vi "Read Transconductance (Voltage).vi"(0 "VISA resource name":refnum<visa-resource-name>, 1 "Pulse Stop Level (0.1 V)":dbl=0.1, 2 "Pulse Start Level (0 V)":dbl, 5 "Source Measure Unit Channel (0: Channel A)":i32(ring) items=["Channel A", "Channel B"], 7 "Current Buffer (ibuffer)":string="ibuffer", 9 "Voltage Buffer (vbuffer)":string="vbuffer", 11 "error in (no error)":errorcluster, 12 "Pulse Measure Cycles (10)":i32=10) -> (4 "VISA resource name out":refnum<visa-resource-name>, 6 "Transconductance":dbl[](array[numeric]), 8 "Current (A)":dbl[](array[numeric]), 10 "Voltage (V)":dbl[](array[numeric]), 15 "error out":errorcluster)   [LabVIEW 2015, in "Keithley 2600 Series.lvlib"]
doc: "Performs a linear voltage sweep and calculates the transconductance.\n\n<b>Note:</b>\nThere are three options for the measurements during the voltage sweep: transconductance measurement; transconductance and current measurement; transconductance, voltage and current measurement."
uses:
  Keithley 2600 Series.lvlib
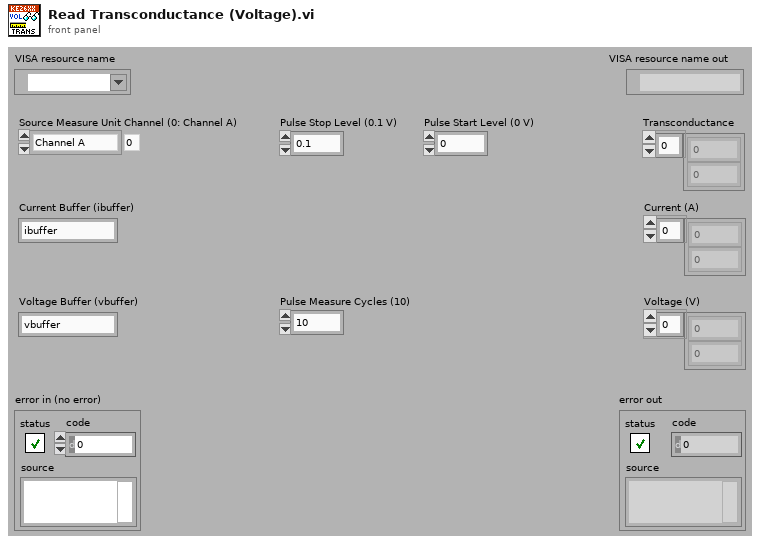
[diagram p1: front panel]
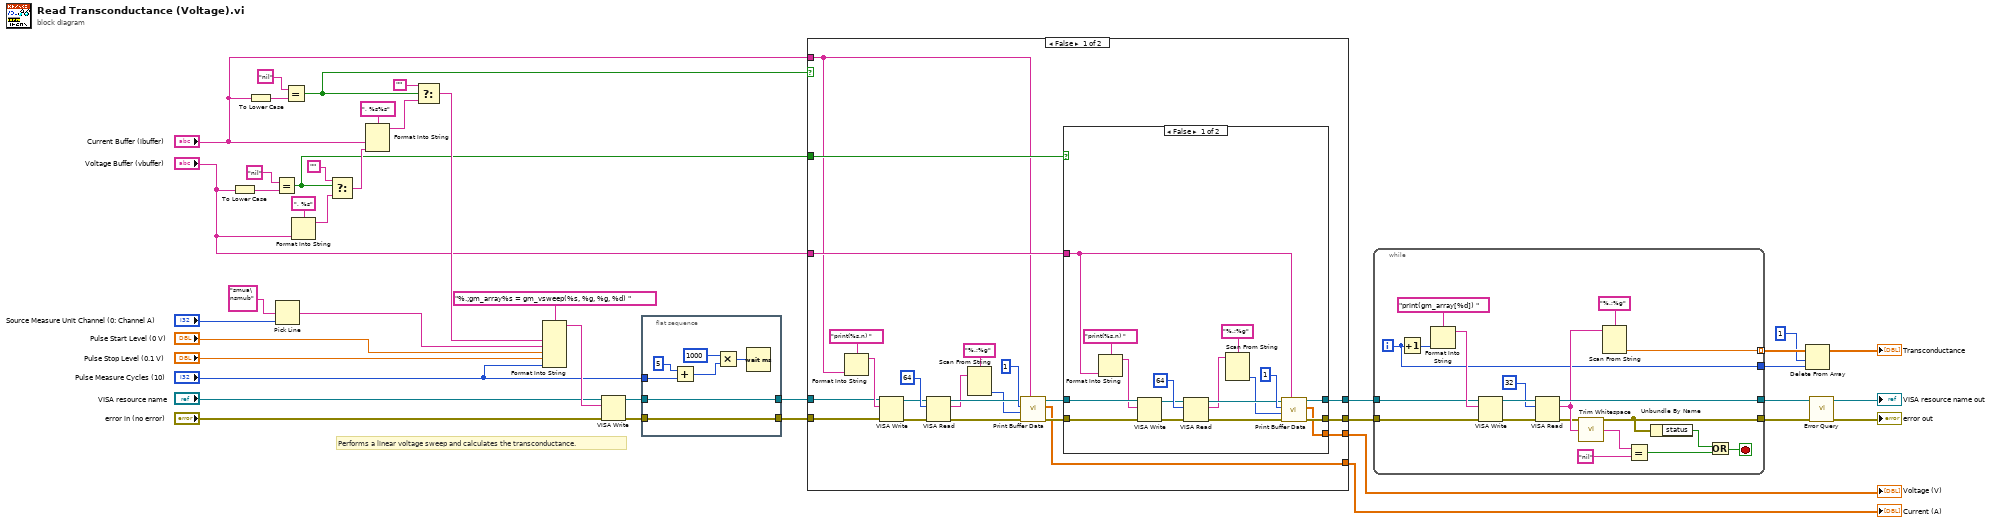
[diagram p0: block diagram]
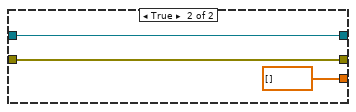
[diagram p2: hidden frame]
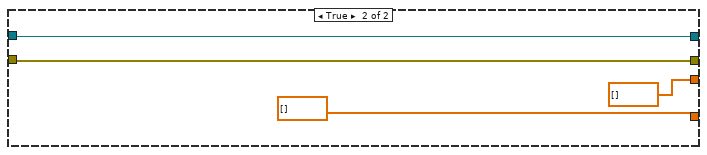
[diagram p3: hidden frame]
diagram:
  # "Performs a linear voltage sweep and calculates the transconductance."
  n1 = To Lower Case(string="Voltage Buffer (vbuffer)") -> (all lower case string=w7:string)
  n2 = To Lower Case(string="Current Buffer (ibuffer)") -> (all lower case string=w9:string)
  n3 = Equal?(x="nil", y=w7) -> (x = y?=w27:bool)
  n4 = Pick Line(multi-line string="smua\nsmub", line index="Source Measure Unit Channel (0: Channel A)") -> (output string=w29:string)  [unwired: 1 in]
  n5 = Equal?(x="nil", y=w9) -> (x = y?=w28:bool)
  n6 = Format Into String(format string=", %s", "Voltage Buffer (vbuffer)") -> (resulting string=w33:string)  [unwired: 2 in, 1 out]
  n7 = Select(t="", s=w27, f=w33) -> (s? t:f=w32:string)
  n8 = Format Into String(format string=", %s%s", "Current Buffer (ibuffer)", w32) -> (resulting string=w31:string)  [unwired: 2 in, 1 out]
  n9 = Select(t="", s=w28, f=w31) -> (s? t:f=w30:string)
  n10 = Format Into String(format string="%.;gm_array%s = gm_vsweep(%s, %g, %g, %d) ", w30, w29, "Pulse Start Level (0 V)", "Pulse Stop Level (0.1 V)", "Pulse Measure Cycles (10)") -> (resulting string=w41:string)  [unwired: 2 in, 1 out]
  n11 = VISA Write(VISA resource name="VISA resource name", write buffer=w41, error in (no error)="error in (no error)") -> (VISA resource name out=w13:refnum<visa-resource-name>, error out=w12:errorcluster)  [unwired: 1 out]
  n12 = flat-sequence {
    tunnel: w13 -> [w49]
    tunnel: w12 -> [w48]
    tunnel: [w49] -> w11
    tunnel: [w48] -> w10
    tunnel: "Pulse Measure Cycles (10)" -> [w46]
    frame #0 {
      n13 = Add(x=5, y=w46) -> (x+y=w44:i32)
      n14 = Multiply(x=1000 ("y"), y=w44) -> (x*y=w43:i32)
      n15 = Wait (ms)(milliseconds to wait=w43) -> ()  [unwired: 1 out]
    }
  }
  n16 = case shown="False" w28 {
    tunnel: [w56 w95] -> w26
    tunnel: w11 -> [w60 w95]
    tunnel: w10 -> [w59 w94]
    tunnel: [w55 w94] -> w25
    tunnel: w27 -> [w54 _]
    tunnel: "Voltage Buffer (vbuffer)" -> [w53 _]
    tunnel: [w52 dbl[] [] ("Buffer Data")] -> w15
    tunnel: [w51 dbl[] [] ("Buffer Data")] -> w14
    tunnel: "Current Buffer (ibuffer)" -> [w50 _]
    frame False {
      n17 = Format Into String(format string="print(%s.n) ", w50) -> (resulting string=w61:string)  [unwired: 2 in, 1 out]
      n18 = VISA Write(VISA resource name=w60, write buffer=w61, error in (no error)=w59) -> (VISA resource name out=w64:refnum<visa-resource-name>, error out=w63:errorcluster)  [unwired: 1 out]
      n19 = VISA Read(VISA resource name=w64, byte count=u32 64, error in (no error)=w63) -> (VISA resource name out=w69:refnum<visa-resource-name>, read buffer=w67:string, error out=w68:errorcluster)  [unwired: 1 out]
      n20 = Scan From String(format string="%.;%g", input string=w67) -> (output 1=w66:i32)  [unwired: 3 in, 3 out]
      n21 = call "Print Buffer Data.vi"("Reading Buffer (smua.nvbuffer1)"=w50, "error in (no error)"=w68, "End Index (1)"=w66, "Start Index (1)"=1 ("Start Index (0)"), "VISA resource name"=w69) -> ("error out"=w57:errorcluster, "Buffer Data"=w52:dbl[], "VISA resource name out"=w58:refnum<visa-resource-name>)  [unwired: 4 in]
      n22 = case shown="False" w54 {
        tunnel: w58 -> [w80 w91]
        tunnel: w57 -> [w79 w90]
        tunnel: [w78 w91] -> w56
        tunnel: [w77 w90] -> w55
        tunnel: w53 -> [w74 _]
        tunnel: [w73 dbl[] [] ("Buffer Data")] -> w51
        frame False {
          n23 = Format Into String(format string="print(%s.n) ", w74) -> (resulting string=w75:string)  [unwired: 2 in, 1 out]
          n24 = VISA Write(VISA resource name=w80, write buffer=w75, error in (no error)=w79) -> (VISA resource name out=w82:refnum<visa-resource-name>, error out=w81:errorcluster)  [unwired: 1 out]
          n25 = VISA Read(VISA resource name=w82, byte count=u32 64, error in (no error)=w81) -> (VISA resource name out=w86:refnum<visa-resource-name>, read buffer=w84:string, error out=w85:errorcluster)  [unwired: 1 out]
          n26 = Scan From String(format string="%.;%g", input string=w84) -> (output 1=w83:i32)  [unwired: 3 in, 3 out]
          n27 = call "Print Buffer Data.vi"("Reading Buffer (smua.nvbuffer1)"=w74, "error in (no error)"=w85, "End Index (1)"=w83, "Start Index (1)"=1 ("Start Index (0)"), "VISA resource name"=w86) -> ("error out"=w77:errorcluster, "Buffer Data"=w73:dbl[], "VISA resource name out"=w78:refnum<visa-resource-name>)  [unwired: 4 in]
        }
        frame True {
        }
      }
    }
    frame True {
    }
  }
  "Voltage (V)" <- w14
  "Current (A)" <- w15
  n28 = while {
    tunnel: w26 -> [w111]
    tunnel: w25 -> [w110]
    tunnel: [w107] -> w24
    tunnel: [w99] -> w23
    tunnel: [w101] -> w5 mode=indexing
    tunnel: [w100] -> w3
    i -> [w100]
    stop <- w98 stop-if-true
    n29 = Increment(x=w100) -> (x+1=w114:i32)
    n30 = Format Into String(format string="print(gm_array[%d]) ", w114) -> (resulting string=w112:string)  [unwired: 2 in, 1 out]
    n31 = VISA Write(VISA resource name=w111, write buffer=w112, error in (no error)=w110) -> (VISA resource name out=w109:refnum<visa-resource-name>, error out=w108:errorcluster)  [unwired: 1 out]
    n32 = VISA Read(VISA resource name=w109, byte count=u32 32, error in (no error)=w108) -> (VISA resource name out=w107:refnum<visa-resource-name>, read buffer=w103:string, error out=w99:errorcluster)  [unwired: 1 out]
    n33 = call <vilib>:"Trim Whitespace.vi"("string"=w103) -> ("trimmed string"=w104:string)  [unwired: 1 in]
    n34 = Scan From String(format string="%.;%g", input string=w103) -> (output 1=w101:dbl)  [unwired: 3 in, 3 out]
    n35 = Equal?(x=w104, y="nil") -> (x = y?=w96:bool)
    n36 = Unbundle By Name(w99) -> ("status"=w97:bool)
    n37 = Or(x=w97, y=w96) -> (x .or. y?=w98:bool)
  }
  n38 = Delete From Array(array=w5, length=1, index=w3) -> (array with subset deleted=→"Transconductance":dbl[])  [unwired: 1 out]
  n39 = call "Error Query.vi"("error in (no error)"=w23, "VISA resource name"=w24) -> ("error out"=→"error out":errorcluster, "VISA resource name out"=→"VISA resource name out":refnum<visa-resource-name>)  [unwired: 6 in, 2 out]
